vi "Distancie_To_Move.vi"(0 "Set-Point X":i32, 1 "Set-Point Y":i32, 2 "Set-Point Z":i32, 3 "Posicion X":i32, 4 "Posicion Y":i32, 5 "Posicion Z":i32) -> (14 "resulting string":string)   [LabVIEW 2021]
panel:
  out "x-y 3":i32
  out "x-y 2":i32
  out "x-y":i32
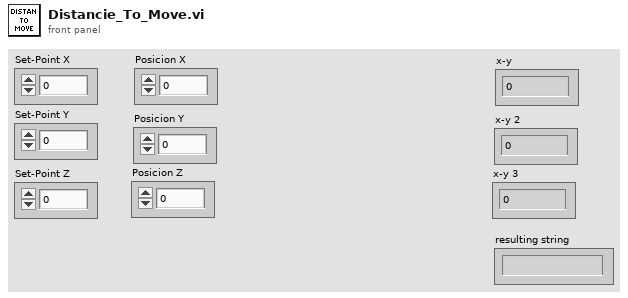
[diagram p1: front panel]
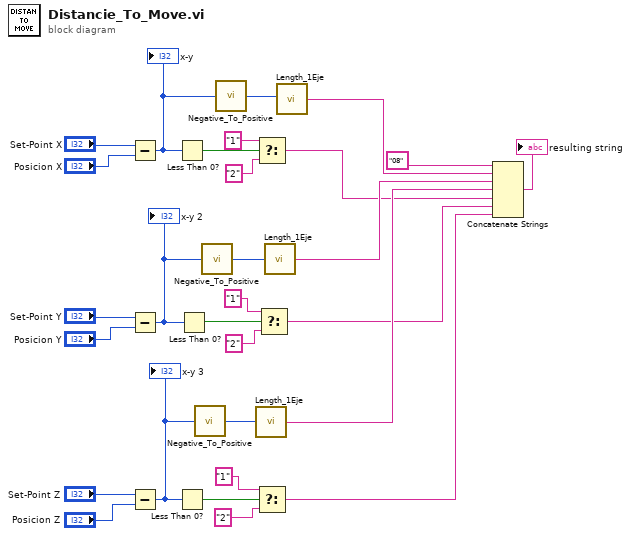
[diagram p0: block diagram]
diagram:
  n1 = Subtract(x="Set-Point X", y="Posicion X") -> (x-y=w5:i32)
  "x-y" <- w5
  n2 = Subtract(x="Set-Point Y", y="Posicion Y") -> (x-y=w3:i32)
  "x-y 2" <- w3
  n3 = Subtract(x="Set-Point Z", y="Posicion Z") -> (x-y=w1:i32)
  "x-y 3" <- w1
  n4 = Less Than 0?(x=w5) -> (x < 0?=w23:bool)
  n5 = Less Than 0?(x=w1) -> (x < 0?=w21:bool)
  n6 = Less Than 0?(x=w3) -> (x < 0?=w22:bool)
  n7 = call "Negative_To_Positive.vi"("Number"=w1) -> ("Positive"=w2:i32)
  n8 = call "Negative_To_Positive.vi"("Number"=w3) -> ("Positive"=w4:i32)
  n9 = call "Negative_To_Positive.vi"("Number"=w5) -> ("Positive"=w6:i32)
  n10 = call "Length_1Eje.vi"("Dist_Eje"=w2) -> ("Dist_EjeSTR"=w10:string)
  n11 = Select(t="1", s=w23, f="2") -> (s? t:f=w9:string)
  n12 = Select(t="1", s=w21, f="2") -> (s? t:f=w7:string)
  n13 = Select(t="1", s=w22, f="2") -> (s? t:f=w8:string)
  n14 = call "Length_1Eje.vi"("Dist_Eje"=w4) -> ("Dist_EjeSTR"=w11:string)
  n15 = call "Length_1Eje.vi"("Dist_Eje"=w6) -> ("Dist_EjeSTR"=w12:string)
  n16 = Concatenate Strings("08", w12, w11, w10, w9, w8, w7) -> (→"resulting string":string)
